vi "EvtFromIni.vi"(8 "ErrorArray In":errorcluster[](array[cluster]), 10 "PathToIni":path, 11 "Bus in":refnum<class "Bus.lvclass">) -> (0 "ErrorArray Out":errorcluster[](array[cluster]), 3 "Bus out":refnum<class "Bus.lvclass">)   [LabVIEW 2017, in "Bus_class.lvlib" / "Bus.lvclass"]
uses:
  Bus.lvclass
  Init/TypeDefs/clInitParams.ctl
  Public/TypeDefs/clBusData.ctl
  FrontPanel/TypeDefs/clEventConfig.ctl
  Modules/PmuImpairPlugins/PmuImpairPluginBase_class/TypeDefs/clImpairConfig.ctl
  Modules/EventPlugins/EventPluginBaseClass/TypeDefs/clEvtReportArray.ctl
  Modules/EventPlugins/EventPluginBaseClass/TypeDefs/clEvtReport.ctl
  Modules/EventPlugins/EventPluginBaseClass/TypeDefs/dblEvtSignalArray.ctl
  Modules/NetworkImpairmentModule/PublicAPI/Arguments/Broadcasts/dblNetworkTime.ctl
  Modules/NetworkImpairmentModule/PublicAPI/Arguments/Broadcasts/dblPktLoss.ctl
  Modules/FlagImpairModule/PublicAPI/Arguments/Broadcasts/ui32FlagImpairmentArray.ctl
  Modules/OutputToFilePlugins/OutputToFileBasePlugin/Typedefs/PmuCfgOpt.ctl
  <vilib>/Utility/config.llb/NI_LVConfig.lvlib
  Framework.lvlib
  Modules/PmuImpairPlugins/PmuImpairPluginBase_class/PmuImpairPluginBase.lvclass
  Modules/EventPlugins/EventPluginBaseClass/EventPluginBaseClass.lvclass
  Modules/NetworkImpairmentModule/NetworkImpairmentModule.lvlib
  Modules/FlagImpairModule/FlagImpairModule.lvlib
  Modules/OutputToFilePlugins/OutputToFileBasePlugin/OutputToFileBasePlugin.lvclass
  <userlib>/NIST/NISTErrorLib/NISTErrorLib.lvlib
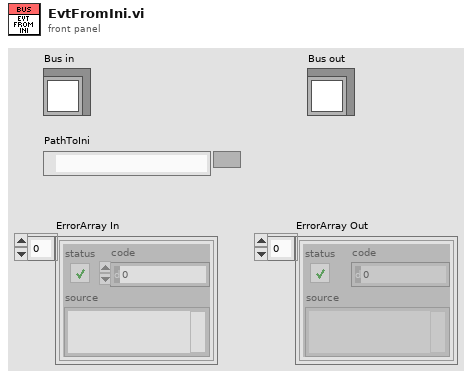
[diagram p1: front panel]
types:
  T1 = typedef "Bus_class.lvlib/Bus.lvclass/clBusData.ctl" = cluster{"BusNumber":u8, "EvtPluginINIFilePath":path, "EvtParams":string[][], "EvtConfig":T2, "Start Time":dbl, "End Time":dbl, "PmuImpairPluginINIFilePath":path, "PmuImpairParams ":string[][], "PmuImpairConfig":T3, "NetImpPluginINIFilePath":path, "NetImpParams":string[][], "FlagImpPluginINIFilePath":path, "FlagImpParams":string[][], "EvtReportArray":T4, "EventSignalArray":T6, "ImpairReportArray":T4, "NetworkTime":T7, "PktLoss":T8, "FlagImpArray":T9, "OutputToFilePluginINIFilePath":path, "Output File Path":path, "clConfigOptions":T10, "AppPluginINIFilePath":path, "AppConfig":variant, "AppOutput":variant}
  T2 = typedef "Framework.lvlib/clEventConfig.ctl" = cluster{"UTC Time 0":timestamp, "Nominal Frequency":u16, "Reporting Rate":u16, "Fsamp":u32, "PosSeq":bool}
  T3 = typedef "PmuImpairPlugins.lvlib/PmuImpairPluginBase.lvclass/clImpairConfig.ctl" = cluster{"FilterType":string, "bPosSeq":bool}
  T4 = typedef "EventPlugins.lvlib/EventPluginBaseClass.lvclass/clEvtReportArray.ctl" = T5[]
  T5 = typedef "EventPlugins.lvlib/EventPluginBaseClass.lvclass/clEvtReport.ctl" = cluster{"Timestamp":dbl, "Synx":cdb[], "Freq":dbl, "ROCOF":dbl, "ID":i16}
  T6 = typedef "EventPlugins.lvlib/EventPluginBaseClass.lvclass/dblEvtSignalArray.ctl" = dbl[][]
  T7 = typedef "NetworkImpairmentModule.lvlib/dblNetworkTime.ctl" = dbl[]
  T8 = typedef "NetworkImpairmentModule.lvlib/dblPktLoss.ctl" = dbl[]
  T9 = typedef "FlagImpairModule.lvlib/ui32FlagImpairmentArray.ctl" = u32[]
  T10 = typedef "OutputToFilePlugins.lvlib/OutputToFileBasePlugin.lvclass/PmuCfgOpt.ctl" = cluster{"TIME_BASE":u64, "STN":string, "IDCODE":u16, "rdoPolRect":enum32{"Rectangular", "Polar"}, "rdoFloatInt":enum32{"Float", "Integer"}, "PHUNIT":u64, "rdoFreqDfreq":enum32{"Float", "Integer"}, "CHNAM":string[], "chkCfg2Prefix":bool}
  T11 = typedef "Framework.lvlib/clInitParams.ctl" = cluster{"RowHdrs":string[], "ColHdrs":string[], "DefaultParams":string[][]}
  T12 = typedef "NI_LVConfig.lvlib/Config Data RefNum.ctl" = refnum<k1>
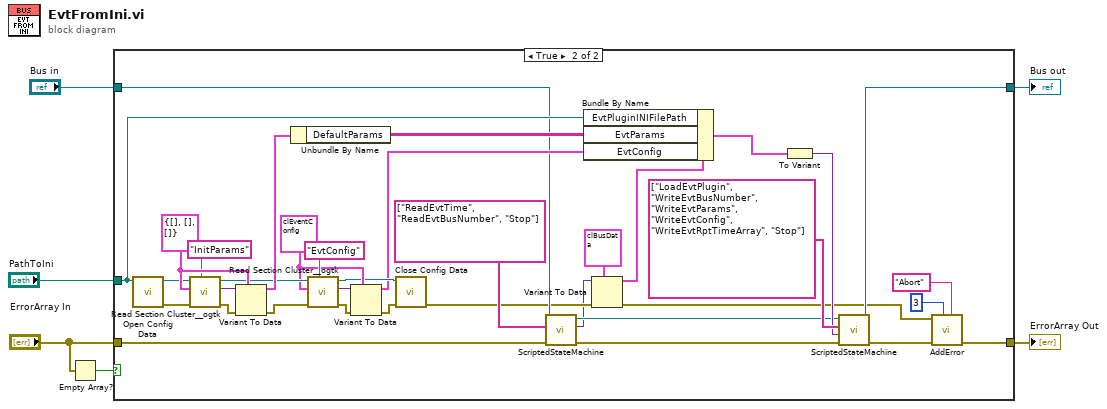
[diagram p0: block diagram]
diagram:
  n1 = Empty Array?(array="ErrorArray In") -> (empty?=w5:bool)
  n2 = case shown="True" w5 {
    tunnel: "ErrorArray In" -> [w8 w22]
    tunnel: [w8 w12] -> w4
    tunnel: "Bus in" -> [w7 w19]
    tunnel: [w7 w23] -> w2
    tunnel: "PathToIni" -> [_ w27]
    frame False {
    }
    frame True {
      w32 = T2 {"UTC Time 0"=timestamp(0 s since 1904-01-01), "Nominal Frequency"=60, "Reporting Rate"=60, "Fsamp"=960, "PosSeq"=FALSE} ("EvtConfig")
      w44 = T11 {"RowHdrs"=[], "ColHdrs"=[], "DefaultParams"=[]} ("ParamsHdrs")
      n3 = call <vilib>:"Open Config Data.vi"("configuration file path"=w27) -> ("error out"=w39:errorcluster, "refnum"=w40:T12)  [unwired: 8 in, 1 out]
      n4 = call <userlib>:"Read Section Cluster__ogtk.vi"("section (optional)"="InitParams", "error in (no error)"=w39, "Section Formatted Cluster Type"=w44, "refnum"=w40) -> ("error out"=w42:errorcluster, "Section Formatted Cluster"=w43:variant, "dup refnum"=w36:T12)  [unwired: 3 in, 2 out]
      n5 = Variant To Data(error in=w42, type=w44, Variant=w43) -> (data=w38:T11, error out=w37:errorcluster)
      n6 = Unbundle By Name(w38) -> ("DefaultParams"=w28:string[][])
      n7 = call <userlib>:"Read Section Cluster__ogtk.vi"("section (optional)"="EvtConfig", "error in (no error)"=w37, "Section Formatted Cluster Type"=w32, "refnum"=w36) -> ("error out"=w34:errorcluster, "Section Formatted Cluster"=w33:variant, "dup refnum"=w30:T12)  [unwired: 3 in, 2 out]
      n8 = Variant To Data(error in=w34, type=w32, Variant=w33) -> (data=w29:T2, error out=w31:errorcluster)
      n9 = call <vilib>:"Close Config Data.vi"("error in (no error)"=w31, "refnum"=w30) -> ("error out"=w17:errorcluster)  [unwired: 8 in, 1 out]
      n10 = call "ScriptedStateMachine.vi"("ErrorArray In"=w22, "Script"=string[] ["ReadEvtTime", "ReadEvtBusNumber", "Stop"], "Bus"=w19) -> ("ErrorArray Out"=w21:errorcluster[], "Data out"=w15:variant, "Bus"=w18:refnum<class "Bus.lvclass">)  [unwired: 6 in]
      n11 = Variant To Data(error in=w17, type=T1 {"BusNumber"=0, "EvtPluginINIFilePath"=path "", "EvtParams"=[], "EvtConfig"={"UTC Time 0"=timestamp(0 s since 1904-01-01), "Nominal Frequency"=60, "Reporting Rate"=60, "Fsamp"=960, "PosSeq"=FALSE}, "Start Time"=0.0, "End Time"=0.0, "PmuImpairPluginINIFilePath"=path "", "PmuImpairParams "=[["960"], ["8.19"], ["164"]], "PmuImpairConfig"={"FilterType"="", "bPosSeq"=TRUE}, "NetImpPluginINIFilePath"=path "", "NetImpParams"=[], "FlagImpPluginINIFilePath"=path "", "FlagImpParams"=[], "EvtReportArray"=[], "EventSignalArray"=[], "ImpairReportArray"=[], "NetworkTime"=[], "PktLoss"=[], "FlagImpArray"=[], "OutputToFilePluginINIFilePath"=path "", "Output File Path"=path "", "clConfigOptions"={"TIME_BASE"=1000000, "STN"="Bus_1", "IDCODE"=0, "rdoPolRect"=enum."Rectangular", "rdoFloatInt"=enum."Float", "PHUNIT"=1000000, "rdoFreqDfreq"=enum."Float", "CHNAM"=["VA", "VB", "VC", "V+", "IA", "IB", "IC", "I+"], "chkCfg2Prefix"=TRUE}, "AppPluginINIFilePath"=path "", "AppConfig"=variant, "AppOutput"=variant} ("clBusData"), Variant=w15) -> (data=w14:T1, error out=w9:errorcluster)
      n12 = Bundle By Name(cluster=w14, "EvtPluginINIFilePath"=w27, "EvtParams"=w28, "EvtConfig"=w29) -> (w25:T1)
      n13 = To Variant(anything=w25) -> (Variant=w24:variant)
      n14 = call "ScriptedStateMachine.vi"("ErrorArray In"=w21, "Data in"=w24, "Script"=string[] ["LoadEvtPlugin", "WriteEvtBusNumber", "WriteEvtParams", "WriteEvtConfig", "WriteEvtRptTimeArray", "Stop"], "Bus"=w18) -> ("ErrorArray Out"=w13:errorcluster[], "Bus"=w23:refnum<class "Bus.lvclass">)  [unwired: 5 in, 1 out]
      n15 = call <userlib>:"AddError.vi"("Severity"="Abort", "Priority"=u8 3, "ErrorArray"=w13, "error in (no error)"=w9) -> ("ErrorArray"=w12:errorcluster[])  [unwired: 6 in, 1 out]
    }
  }
  "ErrorArray Out" <- w4
  "Bus out" <- w2
